vi "Get Cal Point.vi"(0 "Netway":i32, 1 "Init Mean":bool, 5 "Channel to Cal":T1, 7 "Cal Unit":T2, 9 "In/Out":T3, 11 "DMM Connected in":bool, 12 "avg":i32) -> (4 "DMM Connected out":bool, 6 "Output Reading":bool, 8 "Reading":dbl)   [LabVIEW 2013]
uses:
  <vilib>/ptbypt/NI_PtbyPt.lvlib
  Type Defs/Input or Output Type Def.ctl
  Type Defs/Units Type Def (Netway).ctl
  Type Defs/Channel Type Def (Netway).ctl
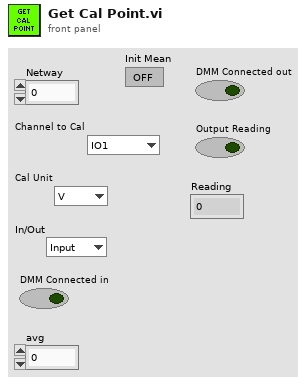
[diagram p1: front panel]
types:
  T1 = typedef "Channel Type Def (Netway).ctl" = enum16{"IO1", "IO2", "IO3", "IO4", "IO5", "IO6", "IO7", "IO8", "IO9", "IO10", "IO11", "IO12", "AIO1", "AIO2", "AIO3", "AIO4", "AIO5", "AIO6", "AIO7", "AIO8"}
  T2 = typedef "Units Type Def (Netway).ctl" = enum16{"V", "%", "Hz"}
  T3 = typedef "Input or Output Type Def.ctl" = enum16{"Input", "Output"}
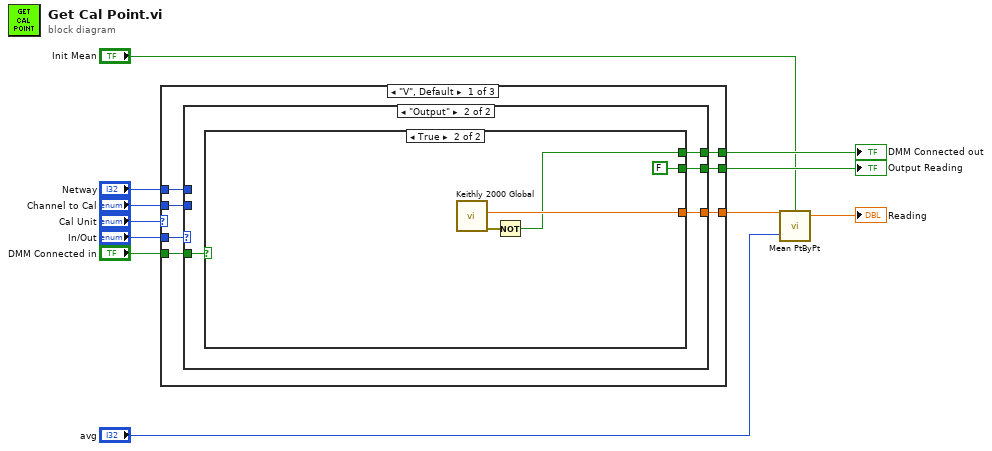
[diagram p0: block diagram]
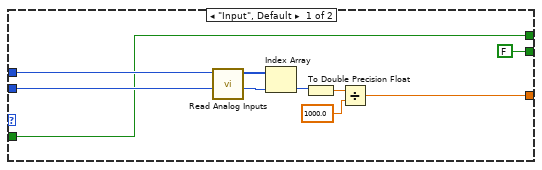
[diagram p2: hidden frame]
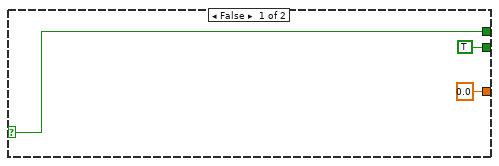
[diagram p3: hidden frame]
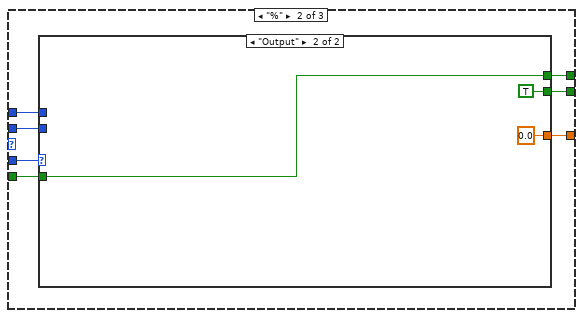
[diagram p4: hidden frame]
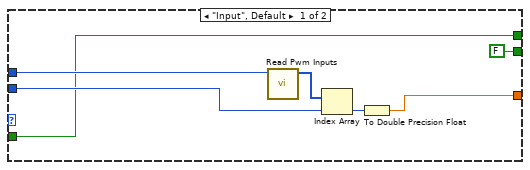
[diagram p5: hidden frame]
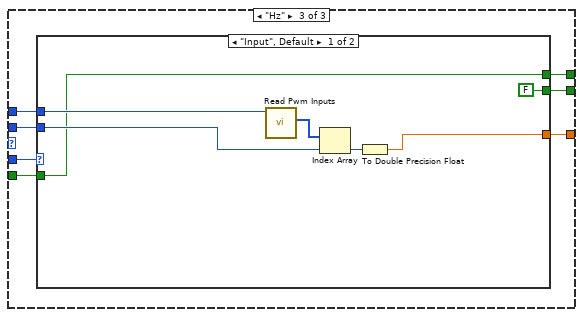
[diagram p6: hidden frame]
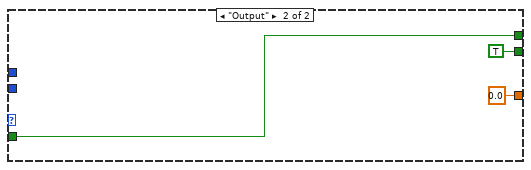
[diagram p7: hidden frame]
diagram:
  n1 = case shown="\"V\", Default" "Cal Unit" {
    tunnel: "Netway" -> [w18 w45 w62]
    tunnel: "Channel to Cal" -> [w17 w44 w61]
    tunnel: [w16 w43 w60] -> w2
    tunnel: "In/Out" -> [w15 w42 w59]
    tunnel: "DMM Connected in" -> [w14 w39 w56]
    tunnel: [w13 w41 w58] -> w10
    tunnel: [w12 w40 w57] -> w11
    frame "V", Default {
      n2 = case shown="\"Output\"" w15 {
        tunnel: w18 -> [w27 _]
        tunnel: w17 -> [w25 _]
        tunnel: [w21 w30] -> w16
        tunnel: w14 -> [w19 w31]
        tunnel: [FALSE w29] -> w13
        tunnel: [w19 w28] -> w12
        frame "Input", Default {
          n3 = call "Read Analog Inputs.vi"("Serial Number"=w27) -> ("Values"=w26:i32[])  [unwired: 9 in, 1 out]
          n4 = Index Array(array=w26, index=w25) -> (element=w24:i32)
          n5 = To Double Precision Float(number=w24) -> (double precision float=w23:dbl)
          n6 = Divide(x=w23, y=1000.0) -> (x/y=w21:dbl)
        }
        frame "Output" {
          n7 = case shown="True" w31 {
            selector: w31 -> [w32 _]
            tunnel: [0.0 ("Measurement") w38] -> w30
            tunnel: [TRUE ("Output Reading") FALSE] -> w29
            tunnel: [w32 w36] -> w28
            frame False {
            }
            frame True {
              n8 = call "Keithly 2000 Global.vi"() -> ("error out"=w37:errorcluster, "Measurement"=w38:dbl)  [unwired: 10 in]
              n9 = Not(x=w37) -> (.not. x?=w36:bool)
            }
          }
        }
      }
    }
    frame "%" {
      n10 = case shown="\"Output\"" w42 {
        tunnel: w45 -> [w52 _]
        tunnel: w44 -> [w50 _]
        tunnel: [w48 0.0] -> w43
        tunnel: [FALSE TRUE] -> w41
        tunnel: [w47 w53] -> w40
        tunnel: w39 -> [w47 w53]
        frame "Input", Default {
          n11 = call "Read Pwm Inputs.vi"("Serial Number"=w52) -> ("Duty"=w51:i32[])  [unwired: 8 in, 2 out]
          n12 = Index Array(array=w51, index=w50) -> (element=w49:i32)
          n13 = To Double Precision Float(number=w49) -> (double precision float=w48:dbl)
        }
        frame "Output" {
        }
      }
    }
    frame "Hz" {
      n14 = case shown="\"Input\", Default" w59 {
        tunnel: w62 -> [w69 _]
        tunnel: w61 -> [w68 _]
        tunnel: [w66 0.0] -> w60
        tunnel: [FALSE TRUE] -> w58
        tunnel: [w64 w70] -> w57
        tunnel: w56 -> [w64 w70]
        frame "Input", Default {
          n15 = call "Read Pwm Inputs.vi"("Serial Number"=w69) -> ("Frequency"=w65:i32[])  [unwired: 8 in, 2 out]
          n16 = Index Array(array=w65, index=w68) -> (element=w67:i32)
          n17 = To Double Precision Float(number=w67) -> (double precision float=w66:dbl)
        }
        frame "Output" {
        }
      }
    }
  }
  "DMM Connected out" <- w11
  "Output Reading" <- w10
  n18 = call <vilib>:"Mean PtByPt.vi"("x"=w2, "sample length"="avg", "initialize"="Init Mean") -> ("mean"=→"Reading":dbl)  [unwired: 1 in, 1 out]
